vi "catalog.get_multiple_ingest_progress_v2.vi"(8 "error in":errorcluster, 10 "datasetRid[]":string[](array[string]), 11 "Nominal Client in":refnum<class "Nominal Client.lvclass">) -> (0 "error out":errorcluster, 1 "Additional Details":T1(array[cluster]) {"End Time" format="%<%x %.3X>T"; "Start Time" format="%<%x %.3X>T"}, 2 "Status":string[](array[string]), 3 "Nominal Client out":refnum<class "Nominal Client.lvclass">)   [LabVIEW 2020, in "Nominal Client.lvclass"]
uses:
  Nominal Client.lvclass
  7433fb34-7591-4323-882c-c8caa2b5fb1a.vi
  <vilib>/JDP Science/JSONtext/JSON text to Variant.vi
  <vilib>/LabVIEW Open Source Project/Epoch Date & Time/formatter.iso8601/ISO8601 DateString to Timestamp.vi
  <vilib>/JDP Science/JSONtext/LVClass Serializer/JSONtext LVClass Serializer.lvclass
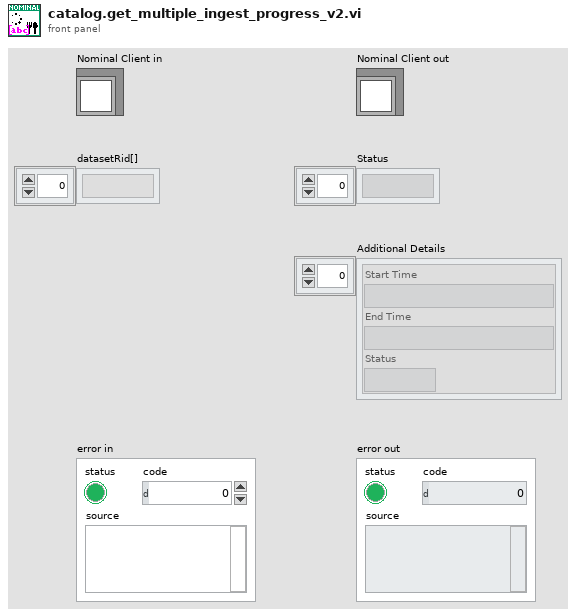
[diagram p1: front panel]
types:
  T1 = cluster{"Start Time":timestamp, "End Time":timestamp, "Status":string}[]
  T2 = cluster{"Start Time":timestamp, "End Time":timestamp, "Status":string}
  T3 = cluster{"startTime":string, "endTime":string, "ingestStatus":cluster{"type":string, "error":cluster{"errorType":string, "message":string}}}
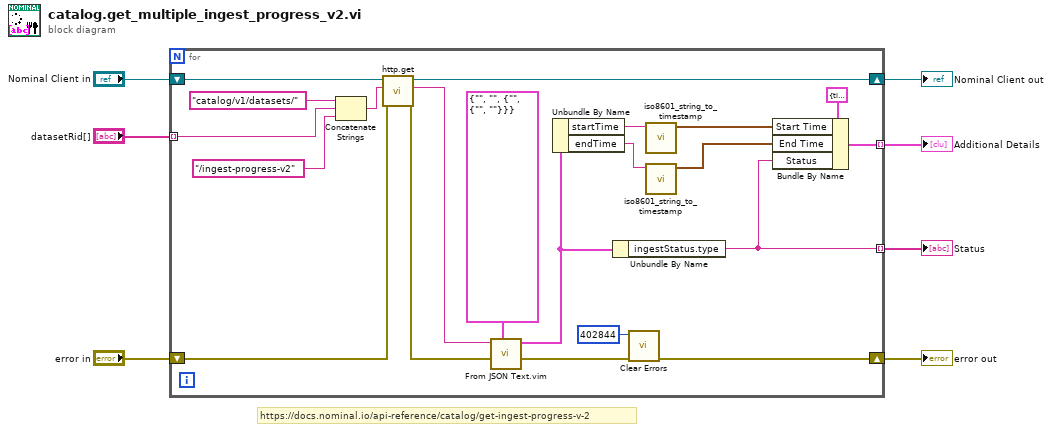
[diagram p0: block diagram]
diagram:
  # "https://docs.nominal.io/api-reference/catalog/get-ingest-progress-v-2"
  n1 = for {
    tunnel: "datasetRid[]" -> [w22] mode=indexing
    tunnel: [w10] -> w2 mode=indexing
    tunnel: [w9] -> w1 mode=indexing
    shift-right: [w27] -> w6
    shift-left: "Nominal Client in" -> [w28]
    shift-right: [w8] -> w3
    shift-left: "error in" -> [w23]
    n2 = Concatenate Strings("catalog/v1/datasets/" ("Path"), w22, "/ingest-progress-v2" ("Path")) -> (w24:string)
    n3 = call "http.get.vi"("error in"=w23, "Path"=w24, "Nominal Client in"=w28) -> ("error out"=w17:errorcluster, "Response"=w18:string, "Nominal Client out"=w27:refnum<class "Nominal Client.lvclass">)  [unwired: 5 in, 1 out]
    n4 = call "From JSON Text.vim"("Data Type and Default Value"=T3 {"startTime"="", "endTime"="", "ingestStatus"={"type"="", "error"={"errorType"="", "message"=""}}}, "error in (no error)"=w17, "JSON"=w18) -> ("error out"=w19:errorcluster, "Data out"=w16:T3)  [unwired: 7 in]
    n5 = Unbundle By Name(w16) -> ("startTime"=w15:string, "endTime"=w14:string)
    n6 = Unbundle By Name(w16) -> ("ingestStatus.type"=w10:string)
    n7 = call <vilib>:"Clear Errors.vi"("error in (no error)"=w19, "specific error code to clear (0: all)"=402844) -> ("error out"=w8:errorcluster)  [unwired: 4 in, 1 out]
    n8 = call "iso8601_string_to_timestamp.vi"("ISO8601 Timestamp String"=w15) -> ("Time Stamp"=w12:timestamp)  [unwired: 9 in, 1 out]
    n9 = call "iso8601_string_to_timestamp.vi"("ISO8601 Timestamp String"=w14) -> ("Time Stamp"=w11:timestamp)  [unwired: 9 in, 1 out]
    n10 = Bundle By Name(cluster=T2 {"Start Time"=timestamp(0 s since 1904-01-01), "End Time"=timestamp(0 s since 1904-01-01), "Status"=""} ("Additional Details"), "Start Time"=w12, "End Time"=w11, "Status"=w10) -> (w9:T2)
  }
  "Nominal Client out" <- w6
  "error out" <- w3
  "Status" <- w2
  "Additional Details" <- w1
